vi "SUM_ARRAY.vi"(7 "Array":string[](array[string])) -> (3 "F-format string":string)   [LabVIEW 2017]
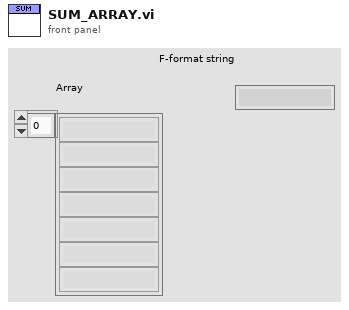
[diagram p1: front panel]
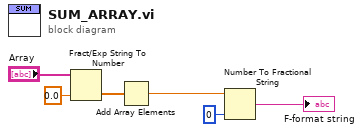
[diagram p0: block diagram]
diagram:
  n1 = Fract/Exp String To Number(string="Array", default (0 dbl)=0.0) -> (number=w6:dbl[])  [unwired: 2 in, 1 out]
  n2 = Add Array Elements(numeric array=w6) -> (sum=w4:dbl)
  n3 = Number To Fractional String(number=w4, precision (6)=i16 0) -> (F-format string=→"F-format string":string)  [unwired: 2 in]
